vi "Omit_Rows_Containing_new.vi"(2 "Data Array In":string[][](array[string]), 3 "Non-Blank Rows":i32[](array[numeric]), 4 "Template Info":string[][](array[string])) -> (0 "Row numbers":i32[](array[numeric]), 1 "Data Array Out":string[][](array[string]))   [LabVIEW 2020]
panel:
  out "No of Rows Removed":i32
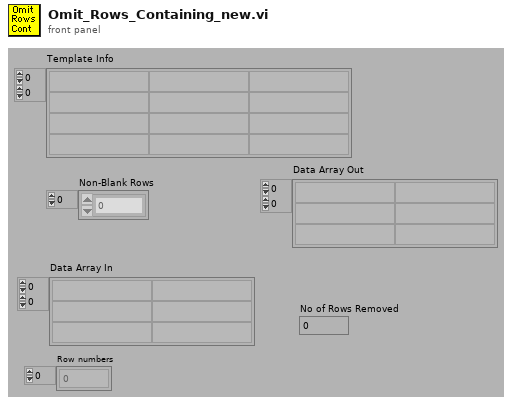
[diagram p1: front panel]
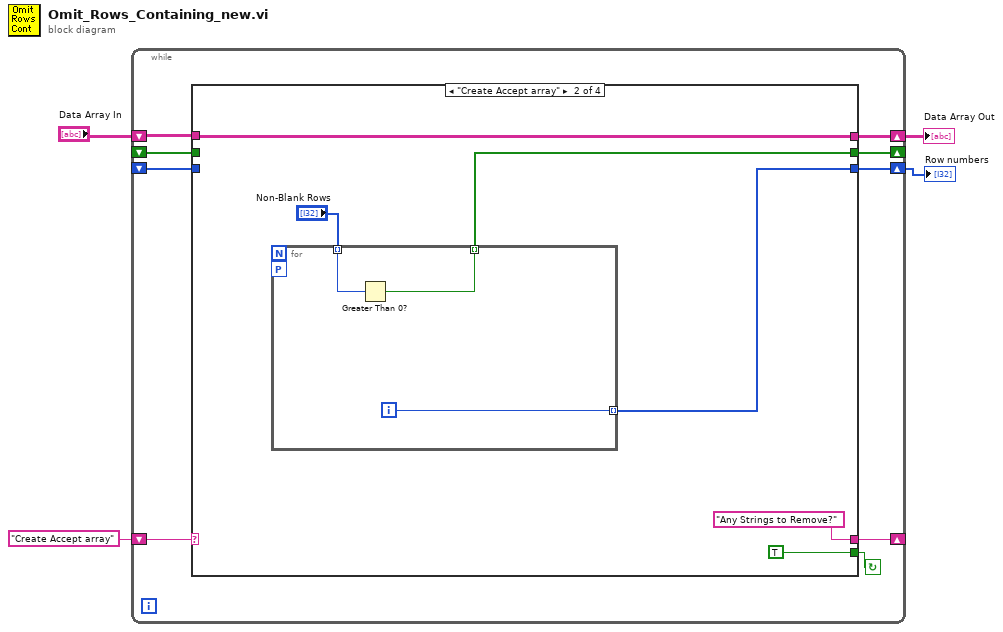
[diagram p0: block diagram]
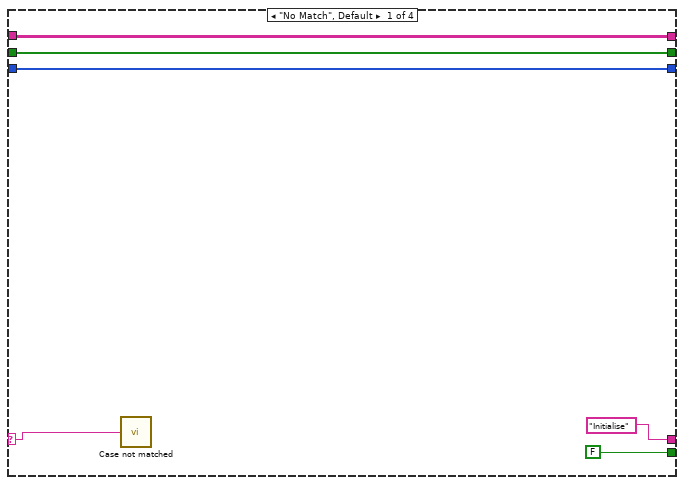
[diagram p2: hidden frame]
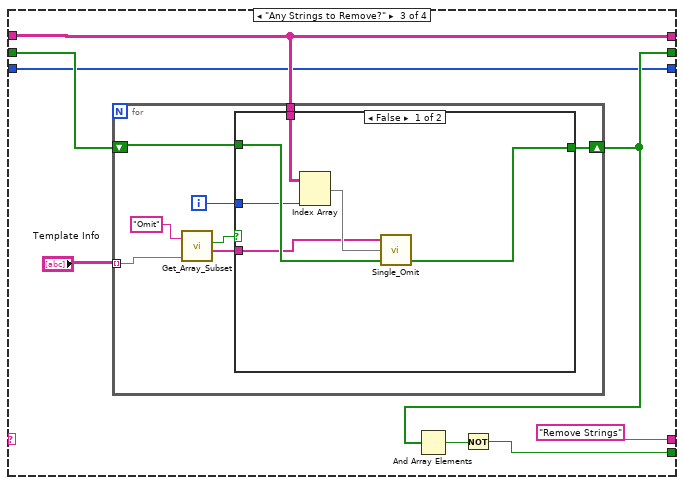
[diagram p3: hidden frame]
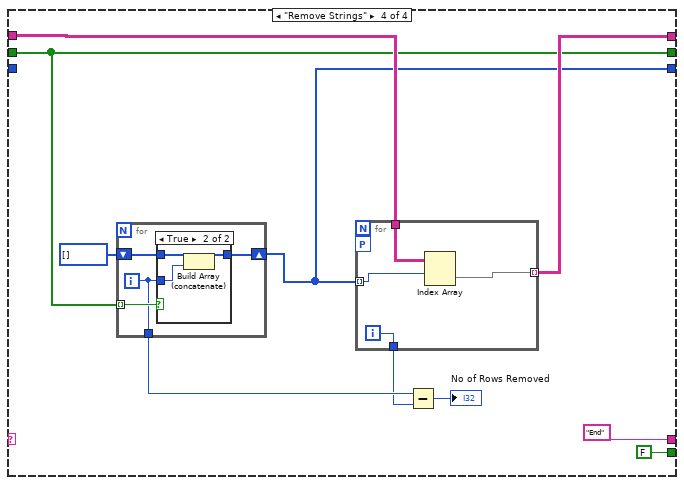
[diagram p5: hidden frame]
diagram:
  n1 = while {
    shift-left: _ -> [w7]
    shift-right: [w8] -> _
    shift-left: "Data Array In" -> [w10]
    shift-right: [w9] -> w2
    shift-left: "Create Accept array" -> [w11]
    shift-right: [w12] -> _
    shift-right: [w6] -> w1
    shift-left: _ -> [w5]
    stop <- w13 continue-if-true
    n2 = case shown="\"Create Accept array\"" w11 {
      selector: w11 -> [w14 _ _ _]
      tunnel: [FALSE TRUE w30 FALSE] -> w13
      tunnel: ["Initialise" "Any Strings to Remove?" "Remove Strings" "End"] -> w12
      tunnel: w10 -> [w17 w21 w33 w59]
      tunnel: [w17 w21 w33 w58] -> w9
      tunnel: [w16 w23 w32 w57] -> w8
      tunnel: w7 -> [w16 _ w34 w57]
      tunnel: [w15 w22 w29 w52] -> w6
      tunnel: w5 -> [w15 _ w29 _]
      frame "No Match", Default {
        n3 = call "Case not matched.vi"("Case Name not Matched"=w14) -> ()
      }
      frame "Create Accept array" {
        n4 = for {
          tunnel: [w26] -> w23 mode=indexing
          tunnel: [w28] -> w22 mode=indexing
          tunnel: "Non-Blank Rows" -> [w27] mode=indexing
          workers-P: _ -> [_]
          i -> [w28]
          n5 = Greater Than 0?(x=w27) -> (x > 0?=w26:bool)
        }
      }
      frame "Any Strings to Remove?" {
        n6 = for {
          tunnel: "Template Info" -> [w43] mode=indexing
          shift-right: [w40] -> w32
          shift-left: w34 -> [w41]
          tunnel: w33 -> [w37]
          i -> [w38]
          n7 = call "Get_Array_Subset.vi"("String Array In"=w43, "Subset Name"="Omit") -> ("Array Subset Out"=w39:string[], "Empty Subset?"=w42:bool)  [unwired: 3 out]
          n8 = case shown="False" w42 {
            tunnel: w41 -> [w50 w51]
            tunnel: [w49 w51] -> w40
            tunnel: w39 -> [w45 _]
            tunnel: w38 -> [w48 _]
            tunnel: w37 -> [w47 _]
            frame False {
              n9 = Index Array(array=w47, index (col)=w48) -> (element=w46:string[])  [unwired: 1 in]
              n10 = call "Single_Omit.vi"("Accept In"=w50, "Data Values"=w46, "Omit Strings"=w45) -> ("Accept Out"=w49:bool[])  [unwired: 2 out]
            }
            frame True {
            }
          }
        }
        n11 = And Array Elements(Boolean array=w32) -> (logical AND=w31:bool)
        n12 = Not(x=w31) -> (.not. x?=w30:bool)
      }
      frame "Remove Strings" {
        n13 = for {
          shift-right: [w68] -> w52
          shift-left: i32[] [] -> [w67]
          tunnel: w57 -> [w69] mode=indexing
          tunnel: [w66] -> w55
          i -> [w66]
          n14 = case shown="True" w69 {
            tunnel: w66 -> [_ w72]
            tunnel: [w70 w71] -> w68
            tunnel: w67 -> [w70 w73]
            frame False {
            }
            frame True {
              n15 = Build Array (concatenate)(w73, w72) -> (w71:i32[])
            }
          }
        }
        n16 = for {
          tunnel: w52 -> [w63] mode=indexing
          tunnel: w59 -> [w65]
          tunnel: [w64] -> w58 mode=indexing
          tunnel: [w62] -> w54
          workers-P: _ -> [_]
          i -> [w62]
          n17 = Index Array(array=w65, index (row)=w63) -> (element=w64:string[])  [unwired: 1 in]
        }
        n18 = Subtract(x=w55, y=w54) -> (x-y=→"No of Rows Removed":i32)
      }
    }
  }
  "Data Array Out" <- w2
  "Row numbers" <- w1
